vi "relativePath.vi"() -> ()   [LabVIEW 2019]
panel:
  out "VI Name":string
  out "path":path
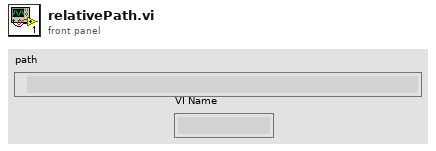
[diagram p1: front panel]
types:
  T1 = enum32{"invalid app kind", "Development System", "Run Time System", "Student Edition", "Embedded LabVIEW", "Evaluation", "Custom"}
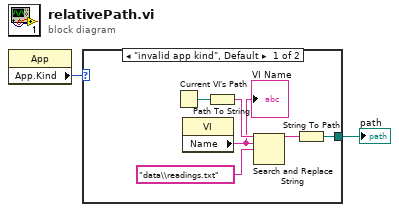
[diagram p0: block diagram]
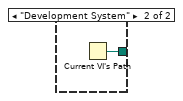
[diagram p2: hidden frame]
diagram:
  n1 = property class="App"() -> ("App.Kind"=w2:T1)  [unwired: 2 in, 2 out]
  n2 = case shown="\"invalid app kind\", Default" w2 {
    tunnel: [w7 w9] -> w1
    frame "invalid app kind", Default {
      n3 = Current VI's Path() -> (path=w4:path)
      n4 = property class="VI"() -> ("Name"=w3:string)  [unwired: 2 in, 2 out]
      "VI Name" <- w3
      n5 = Path To String(path=w4) -> (string=w5:string)
      n6 = Search and Replace String(input string=w5, search string=w3, replace string="data\\readings.txt" ("replace string (\"\")")) -> (result string=w6:string)  [unwired: 5 in, 3 out]
      n7 = String To Path(string=w6) -> (path=w7:path)
    }
    frame "Development System" {
      n8 = Current VI's Path() -> (path=w9:path)
    }
  }
  "path" <- w1
